vi "Protocol.Read J1939 Incoming Messages.vi"(8 "error in (no error)":errorcluster, 11 "J1939 Main Configuration":T1 {"Stream Refs"."Port Settings"."FD ISO Mode" items=["ISO", "Non ISO", "ISO Legacy"]; "Stream Refs"."Port Settings"."Termination" items=["Off", "On"]; "Stream Refs"."Port Settings"."Mode" items=["CAN 2.0", "CAN FD", "CAN FD+BRS"]}) -> (0 "error out":errorcluster)   [LabVIEW 2023, in "J1939 Addon Engine.lvlib"]
uses:
  J1939 Addon Engine.lvlib
  Types/Protocol.Configuration.ctl
  <vilib>/NI/NI VeriStand Addon Network Comm/Engine/VeriStand Comm.lvclass
  <vilib>/NI/NIVS Inline Async API/_VS Inline Async API/Process/Process.lvclass
  Types/Protocol.Refs.ctl
  Support Libraries/J1939 Utilities/Types/CAN Outgoing Message Cluster.ctl
  Types/Protocol.RQST Lookup Table Reference.ctl
  Types/Protocol.Address Table Reference.ctl
  Types/Protocol.XNET Settings.ctl
  <vilib>/NI/NIVS Inline Async API/_Data Access Engine/Data Access Engine/Types/Read.DVR.ctl
  <vilib>/NI/NIVS Inline Async API/_Data Access Engine/Access Type Classes/Read/Read.lvclass
  <vilib>/NI/NIVS Inline Async API/_Data Access Engine/Data Access Engine/Types/Write.DVR.ctl
  <vilib>/NI/NIVS Inline Async API/_Data Access Engine/Access Type Classes/Write/Write.lvclass
  Types/CounterAndProtectionFrames.ctl
  SubModules/Frame-Protection-Support/Source/Engine/Types/RT Frame Settings.ctl
  SubModules/Frame-Protection-Support/Source/Shared/Types/Exported Frame Type.ctl
  SubModules/Frame-Protection-Support/Source/Engine/Types/RT Protection Configuration.ctl
  SubModules/Frame-Protection-Support/Source/Shared/Types/Protection Type.ctl
  SubModules/Frame-Protection-Support/Source/Shared/Types/XNET Signal Configuration.ctl
  SubModules/Frame-Protection-Support/Source/Shared/Types/Exported Counter Settings.ctl
  SubModules/Frame-Protection-Support/Source/Shared/Types/Exported Event Trigger Type.ctl
  SubModules/CAN-Streaming-Support/Source/Addon/Addon Engine/Types/Engine Stream Refs.ctl
  SubModules/CAN-Streaming-Support/Source/Addon/Addon Shared/Types/Direction Filter.ctl
  SubModules/CAN-Streaming-Support/Source/Addon/Addon Shared/Types/Type Filter.ctl
  SubModules/CAN-Streaming-Support/Source/Addon/Addon Shared/Types/Filter Parameters.ctl
  SubModules/CAN-Streaming-Support/Source/Addon/Addon Engine/Types/Engine Stream Port Settings.ctl
  Types/Protocol.RQST Lookup Table Action.ctl
  <vilib>/NI/NIVS Inline Async API/_VS Inline Async API/Process/Process.lvclass/Process.ctl
  Protocol.Process Incoming Messages by PDU F.vi
  Protocol.J1939 Filter by Device Address.vi
  <vilib>/NI/NIVS Inline Async API/_VS Inline Async API/Error Handling Process/SubVIs/Error.ConvertArray.vi
  Support Libraries/J1939 Utilities/Common Conversions.vi
  Support Libraries/J1939 Utilities/SubVIs/Convert CAN Arb ID to J1939 ID.vi
  Protocol.RQST Look for Response.vi
  Support Libraries/J1939 Utilities/SubVIs/Convert J1939 ID to CAN Arb ID.vi
  Support Libraries/J1939 Utilities/SubVIs/Convert CAN Data (U32) to U8.vi
  Protocol.Get Simulated Previously Active DTCs.vi
  Protocol.Get Simulated Active DTCs.vi
  Support Libraries/J1939 Utilities/Common Messages.vi
  Support Libraries/J1939 Utilities/SubVIs/Acknowledgement.vi
  Protocol.Send Reset Previously Active DTC to Main.vi
  Protocol.Send Reset Active DTC to Main.vi
  Protocol.Convert Signals to Frame by ID.vi
  Protocol.Address Lookup Table Action.vi
  Protocol.Parse Message Type.vi
  Protocol.Convert Data to DTC Frame.vi
  <vilib>/xnet/xnet.llb/XNET Read (Frame CAN).vi
  Protocol.RQST Lookup Table.vi
  <vilib>/xnet/xnet.llb/XNET Create Session.vi
  <vilib>/xnet/xnet.llb/XNET Create Session (Conversion).vi
  <vilib>/xnet/xnet.llb/XNET Convert.vi
  <vilib>/xnet/xnet.llb/XNET Convert (Signal to Frame CAN).vi
  <vilib>/xnet/xnet.llb/XNET Clear.vi
  Protocol.Address Lookup Table.vi
  Support Libraries/J1939 Utilities/J1939 Utilities.lvlib
  <vilib>/NI/NIVS Inline Async API/_Data Access Engine/Data Access Engine/Data Access Engine.lvclass
  SubModules/Frame-Protection-Support/Source/Engine/Protection and Counter Support Engine.lvlib
  SubModules/Frame-Protection-Support/Source/Shared/Protection and Counter Support Shared.lvlib
  SubModules/CAN-Streaming-Support/Source/Addon/Addon Shared/CAN Stream Support Shared.lvlib
  SubModules/CAN-Streaming-Support/Source/Addon/Addon Engine/CAN Stream Support Engine.lvlib
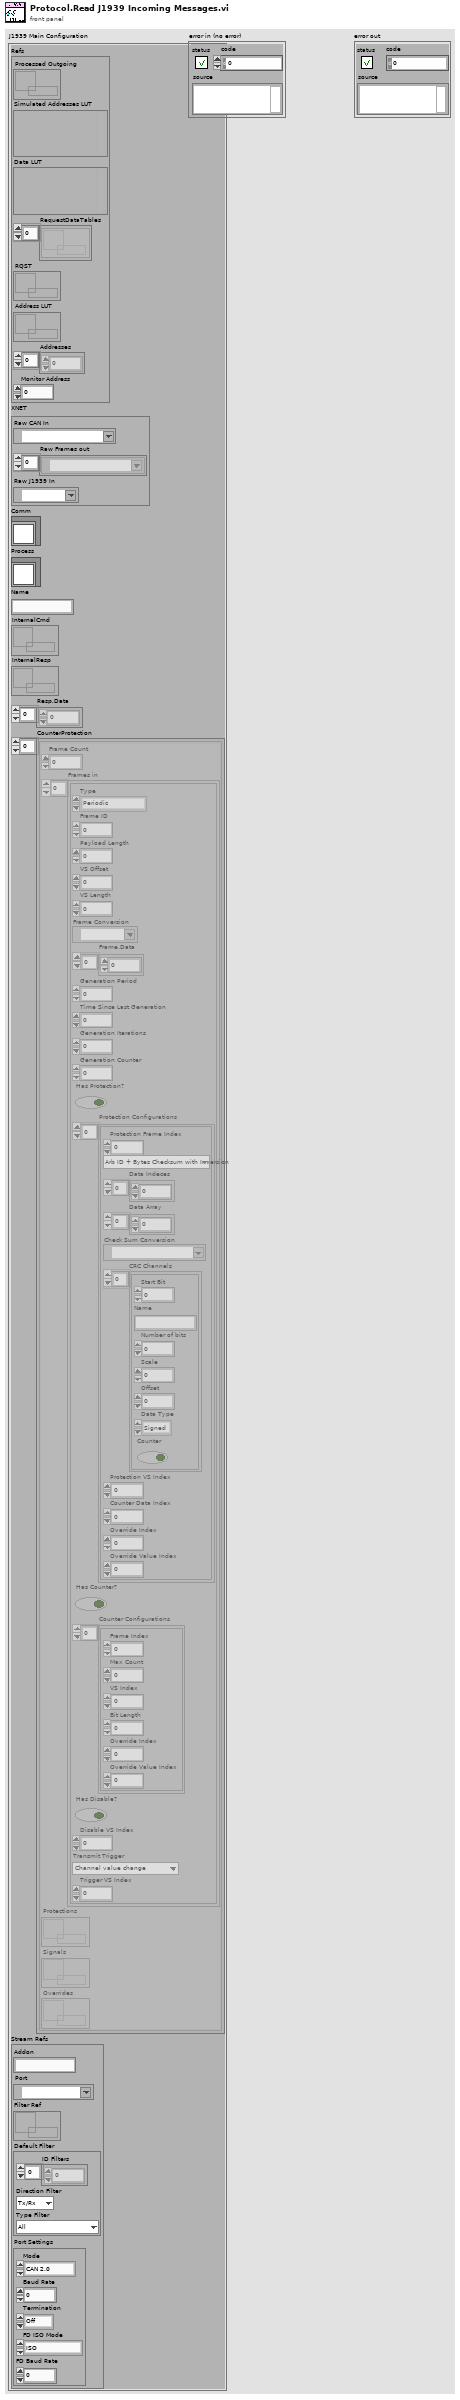
[diagram p1: front panel]
types:
  T1 = typedef "J1939 Addon Engine.lvlib/Protocol.Configuration.ctl" = cluster{"Refs":T2, "XNET":T5, "Comm":refnum<class "VeriStand Comm.lvclass">, "Process":refnum<class "Process.lvclass">, "Name":string, "InternalCmd":T6, "InternalResp":T7, "Resp.Data":dbl[], "CounterProtection":T8[], "Stream Refs":T16}
  T2 = typedef "J1939 Addon Engine.lvlib/Protocol.Refs.ctl" = cluster{"Processed Outgoing":refnum<queue>, "Simulated Addresses LUT":variant, "Data LUT":variant, "RequestDataTables":refnum<k33>[], "RQST":T3, "Address LUT":T4, "Addresses":u8[], "Monitor Address":u8}
  T3 = typedef "J1939 Addon Engine.lvlib/Protocol.RQST Lookup Table Reference.ctl" = refnum<data-value>
  T4 = typedef "J1939 Addon Engine.lvlib/Protocol.Address Table Reference.ctl" = refnum<data-value>
  T5 = typedef "J1939 Addon Engine.lvlib/Protocol.XNET Settings.ctl" = cluster{"Raw CAN In":refnum<k21>, "Raw Frames out":refnum<k21>[], "Raw J1939 In":refnum<k21>}
  T6 = typedef "Data Access Engine.lvlib/Data Access Engine.lvclass/Read.DVR.ctl" = refnum<data-value>
  T7 = typedef "Data Access Engine.lvlib/Data Access Engine.lvclass/Write.DVR.ctl" = refnum<data-value>
  T8 = typedef "J1939 Addon Engine.lvlib/CounterAndProtectionFrames.ctl" = cluster{"Frame Count":i32, "Frames in":T9[], "Protections":T7, "Signals":T6, "Overrides":T6}
  T9 = typedef "Protection and Counter Support Engine.lvlib/RT Frame Settings.ctl" = cluster{"Type":T10, "Frame ID":u32, "Payload Length":u32, "VS Offset":i32, "VS Length":i32, "Frame Conversion":refnum<k21>, "Frame.Data":dbl[], "Generation Period":u32, "Time Since Last Generation":u32, "Generation Iterations":u32, "Generation Counter":u32, "Has Protection?":bool, "Protection Configurations":T11[], "Has Counter?":bool, "Counter Configurations":T14[], "Has Disable?":bool, "Disable VS Index":i32, "Transmit Trigger":T15, "Trigger VS Index":i32}
  T10 = typedef "Protection and Counter Support Shared.lvlib/Exported Frame Type.ctl" = enum16{"Periodic", "Event", "Periodic/Event"}
  T11 = typedef "Protection and Counter Support Engine.lvlib/RT Protection Configuration.ctl" = cluster{"Protection Frame Index":i32, "Protection Type":T12, "Data Indeces":i32[], "Data Array":dbl[], "Check Sum Conversion":refnum<k21>, "CRC Channels":T13[], "Protection VS Index":i32, "Counter Data Index":i32, "Override Index":i32, "Override Value Index":i32}
  T12 = typedef "Protection and Counter Support Shared.lvlib/Protection Type.ctl" = enum16{"Arb ID + Bytes Checksum with Inversion", "Arb ID + Bytes CRC with Inversion", "Reversed Raw Signal Checksum with Inversion", "Concatenated Two's Compliment"}
  T13 = typedef "Protection and Counter Support Shared.lvlib/XNET Signal Configuration.ctl" = cluster{"Start Bit":i32, "Name":string, "Number of bits":i32, "Scale":dbl, "Offset":dbl, "Data Type":u32, "Counter":bool}
  T14 = typedef "Protection and Counter Support Shared.lvlib/Exported Counter Settings.ctl" = cluster{"Frame Index":i32, "Max Count":dbl, "VS Index":i32, "Bit Length":i64, "Override Index":i32, "Override Value Index":i32}
  T15 = typedef "Protection and Counter Support Shared.lvlib/Exported Event Trigger Type.ctl" = enum16{"Channel value change", "Trigger channel (not zero)", "Channel value change or trigger channel (not zero)", "Trigger channel (any value change)", "Channel value change or trigger channel (any value change)"}
  T16 = typedef "CAN Stream Support Engine.lvlib/Engine Stream Refs.ctl" = cluster{"Addon":string, "Port":refnum<k21>, "Filter Ref":refnum<data-value>, "Default Filter":T17, "Port Settings":T20}
  T17 = typedef "CAN Stream Support Shared.lvlib/Filter Parameters.ctl" = cluster{"ID Filters":u32[], "Direction Filter":T18, "Type Filter":T19}
  T18 = typedef "CAN Stream Support Shared.lvlib/Direction Filter.ctl" = enum16{"Tx/Rx", "Rx", "Tx"}
  T19 = typedef "CAN Stream Support Shared.lvlib/Type Filter.ctl" = enum16{"All", "CAN Data", "CAN Remote", "CAN Bus Error", "CAN 2.0 Data", "CAN FD Data", "CAN FD+BRS Data", "J1939 Data", "Delay", "Log Trigger", "Start Trigger"}
  T20 = typedef "CAN Stream Support Engine.lvlib/Engine Stream Port Settings.ctl" = cluster{"Mode":u32, "Baud Rate":u64, "Termination":u32, "FD ISO Mode":u32, "FD Baud Rate":u64}
  T21 = typedef "J1939 Addon Engine.lvlib/Protocol.RQST Lookup Table Action.ctl" = enum16{"Initialize", "Add", "Get", "Remove", "Get Active Requests"}
  T22 = typedef "XNET Frame CAN.ctl" = cluster{"timestamp":timestamp, "payload":u8[], "identifier":u32, "type":T23, "extended?":bool, "echo?":bool}
  T23 = typedef "XNET Frame Type CAN.ctl" = u8
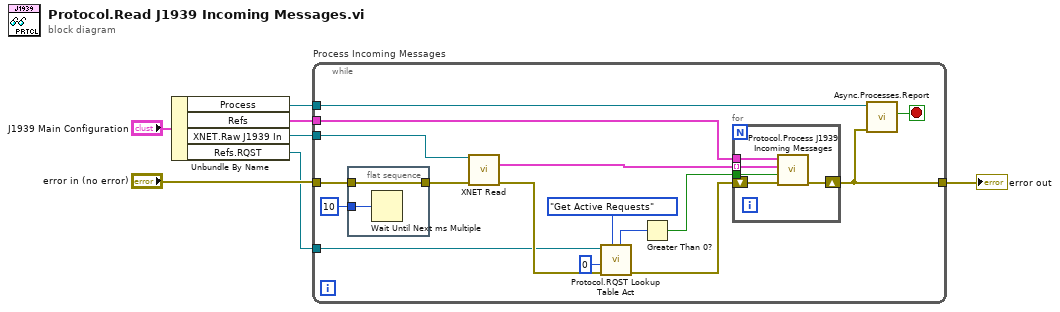
[diagram p0: block diagram]
diagram:
  n1 = Unbundle By Name("J1939 Main Configuration") -> ("Process"=w5:refnum<class "Process.lvclass">, "Refs"=w2:T2, "XNET.Raw J1939 In"=w6:refnum<k21>, "Refs.RQST"=w1:T3)
  n2 = while "Process Incoming Messages" {
    tunnel: w2 -> [w23]
    tunnel: "error in (no error)" -> [w16]
    tunnel: [w12] -> w3
    tunnel: w6 -> [w22]
    tunnel: w5 -> [w14]
    tunnel: w1 -> [w15]
    stop <- w13 stop-if-true
    n3 = flat-sequence {
      tunnel: u32 10 ("Incoming Timeout") -> [w25]
      tunnel: [w24] -> w17
      tunnel: w16 -> [w24]
      frame #0 {
        n4 = Wait Until Next ms Multiple(millisecond multiple=w25) -> ()  [unwired: 1 out]
      }
    }
    n5 = call-poly <vilib>:"XNET Read.vi"("session in"=w22, "error in (no error)"=w17) -> ("data"=w9:T22[], "error out"=w20:errorcluster)  [unwired: 12 out]
    n6 = call "Protocol.RQST Lookup Table Act.vi"("Action"=Protocol.RQST_Lookup_Table_Action."Get Active Requests", "error in (no error)"=w20, "ID"=u32 0, "Rqst LUT"=w15) -> ("error out"=w19:errorcluster, "# of Active Requests"=w10:i32)  [unwired: 3 in, 3 out]
    n7 = Greater Than 0?(x=w10) -> (x > 0?=w18:bool)
    n8 = for {
      tunnel: w9 -> [w26] mode=indexing
      shift-right: [w29] -> w12
      shift-left: w19 -> [w30]
      tunnel: w23 -> [w28]
      tunnel: w18 -> [w27]
      n9 = call "Protocol.Process J1939 Incoming Messages.vi"("error in"=w30, "Active Request?"=w27, "CAN frame"=w26, "J1939 Cluster"=w28) -> ("error out"=w29:errorcluster)  [unwired: 6 in, 1 out]
    }
    n10 = call <vilib>:"Async.Processes.Report.vi"("Error"=w12, "Process in"=w14) -> ("Stop"=w13:bool)  [unwired: 8 in, 1 out]
  }
  "error out" <- w3
